vi "INST_PS_MEAS_WITH_LOOP.vi"(4 "Use OPC?(T)":bool=TRUE, 6 "Instrument Select (Output 1)":string(combo)="OUT1", 7 "Clear Error in":bool, 8 "error in (no error)":errorcluster, 9 "Measurement Type (Voltage)":string(combo)="MEAS:VOLT?", 11 "VISA session":refnum<visa-resource-name>) -> (0 "error out":errorcluster, 2 "Measurement":dbl format="%.2p", 3 "dup VISA session":refnum<visa-resource-name>)   [LabVIEW 2018]
doc: "This VI takes a measurement on the output signal and returns the measured value."
panel:
  in  "Measure\nContinuous":bool
  in  "stop":bool
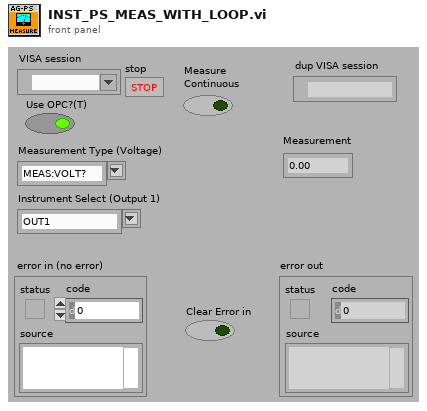
[diagram p1: front panel]
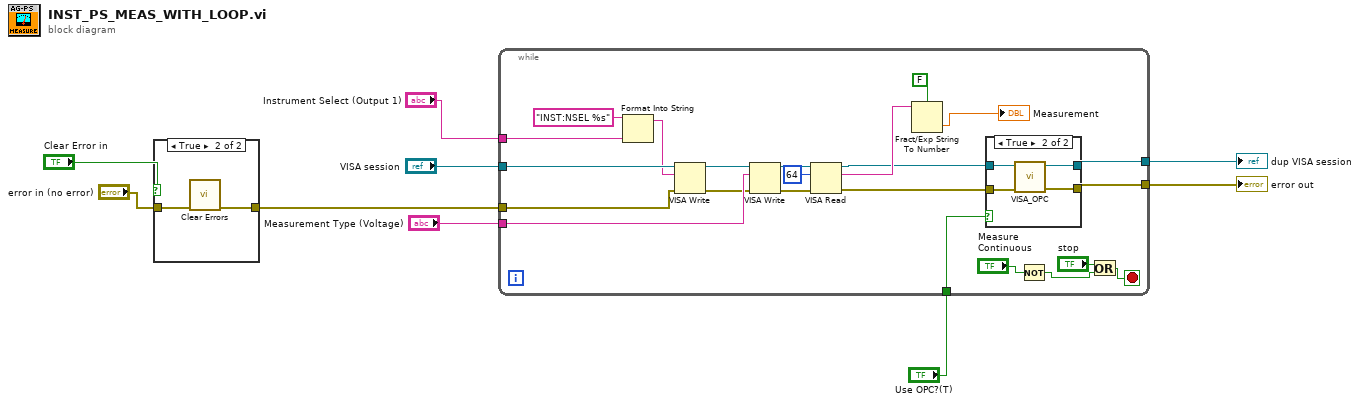
[diagram p0: block diagram]
diagram:
  n1 = case shown="True" "Clear Error in" {
    tunnel: "error in (no error)" -> [w10 w12]
    tunnel: [w10 w11] -> w4
    frame False {
    }
    frame True {
      n2 = call <vilib>:"Clear Errors.vi"("error in (no error)"=w12) -> ("error out"=w11:errorcluster)  [unwired: 5 in, 1 out]
    }
  }
  n3 = while {
    tunnel: "Measurement Type (Voltage)" -> [w35]
    tunnel: "VISA session" -> [w34]
    tunnel: [w33] -> w7
    tunnel: [w32] -> w6
    tunnel: w4 -> [w31]
    tunnel: "Use OPC?(T)" -> [w18]
    tunnel: "Instrument Select (Output 1)" -> [w13]
    stop <- w16 stop-if-true
    n4 = Format Into String(format string="INST:NSEL %s", w13) -> (resulting string=w24:string)  [unwired: 2 in, 1 out]
    n5 = VISA Write(VISA resource name=w34, write buffer=w24, error in (no error)=w31) -> (VISA resource name out=w22:refnum<visa-resource-name>, error out=w23:errorcluster)  [unwired: 1 out]
    n6 = VISA Write(VISA resource name=w22, write buffer=w35, error in (no error)=w23) -> (VISA resource name out=w27:refnum<visa-resource-name>, error out=w30:errorcluster)  [unwired: 1 out]
    n7 = VISA Read(VISA resource name=w27, byte count=u32 64, error in (no error)=w30) -> (VISA resource name out=w20:refnum<visa-resource-name>, read buffer=w28:string, error out=w21:errorcluster)  [unwired: 1 out]
    n8 = Fract/Exp String To Number(use system decimal point (T)=FALSE, string=w28) -> (number=→"Measurement":dbl)  [unwired: 2 in, 1 out]
    n9 = case shown="True" w18 {
      tunnel: w21 -> [w36 w41]
      tunnel: [w36 w40] -> w33
      tunnel: [w37 w39] -> w32
      tunnel: w20 -> [w37 w38]
      frame False {
      }
      frame True {
        n10 = call "VISA_OPC.vi"("error in"=w41, "Session In"=w38) -> ("error out"=w40:errorcluster, "Session Out"=w39:refnum<visa-resource-name>)  [unwired: 7 in, 1 out]
      }
    }
    n11 = Not(x="Measure\nContinuous") -> (.not. x?=w14:bool)
    n12 = Or(x="stop", y=w14) -> (x .or. y?=w16:bool)
  }
  "error out" <- w7
  "dup VISA session" <- w6
